vi "Read Call Chain.vi"(11 "Assert in":refnum<class "Assert.lvclass">) -> (2 "Call Chain":string[](array[string]), 3 "Assert out":refnum<class "Assert.lvclass">)   [LabVIEW 2013, in "Caraya.lvlib" / "Assert.lvclass"]
uses:
  Assert.lvclass
  Assert.lvclass/Assert.ctl
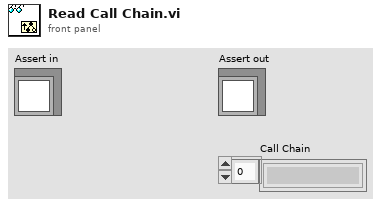
[diagram p1: front panel]
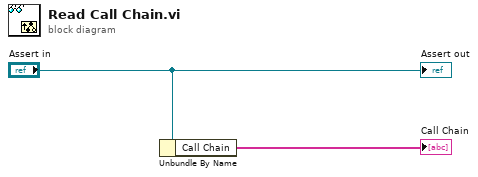
[diagram p0: block diagram]
diagram:
  n1 = Unbundle By Name("Assert in") -> ("Call Chain"=→"Call Chain":string[])
  "Assert out" <- "Assert in"
